vi "Readable String.vi"(11 "OutOfRange Condition in":refnum<class "OutOfRange Condition.lvclass">) -> (2 "String":string)   [LabVIEW 2020, in "VolatusSeq.lvlib" / "OutOfRange Condition.lvclass"]
uses:
  OutOfRange Condition.lvclass
  OutOfRange Condition.lvclass/OutOfRange Condition.ctl
  lv-vecto/Vecto/Channel DBL/Channel DBL.lvclass
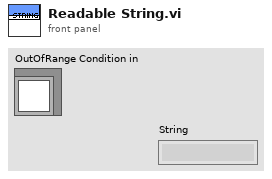
[diagram p1: front panel]
types:
  T1 = typedef "VectoConfig.lvlib/Channel Info.ctl" = cluster{"Name":string, "Group":string, "Owning Node":string, "Owning Task":string, "Resource":string}
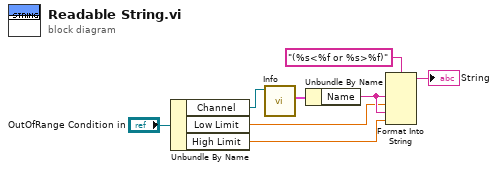
[diagram p0: block diagram]
diagram:
  n1 = Unbundle By Name("OutOfRange Condition in") -> ("Channel"=w7:refnum<class "Channel DBL.lvclass">, "Low Limit"=w3:dbl, "High Limit"=w2:dbl)
  n2 = call "Info.vi"("Channel in"=w7) -> ("Info"=w6:T1)  [unwired: 8 in, 2 out]
  n3 = Unbundle By Name(w6) -> ("Name"=w4:string)
  n4 = Format Into String(format string="(%s<%f or %s>%f)", w4, w3, w4, w2) -> (resulting string=→"String":string)  [unwired: 2 in, 1 out]
